vi "Get mode.vi"() -> (3 "Robot Mode":T1)   [LabVIEW 2011]
uses:
  <vilib>/Rock Robotics/WPI/DriverStation/WPI_DriverStationRobotMode.ctl
  <vilib>/Rock Robotics/WPI/DriverStation/WPI_DriverStationCommDataCacheOp.ctl
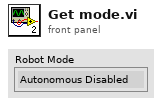
[diagram p1: front panel]
types:
  T1 = typedef "WPI_DriverStationRobotMode.ctl" = enum16{"Autonomous Disabled", "Autonomous Enabled", "Teleop Disabled", "Teleop Enabled", "Timeout", "Finish"}
  T2 = typedef "WPI_DriverStationCommDataCacheOp.ctl" = enum16{"Get", "Set", "Init"}
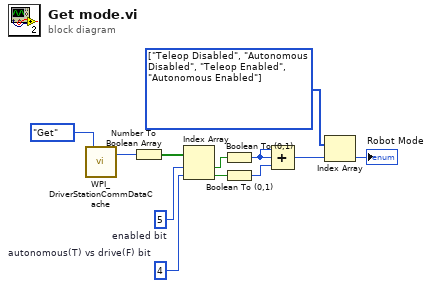
[diagram p0: block diagram]
diagram:
  w7 = T1[] [enum."Teleop Disabled", enum."Autonomous Disabled", enum."Teleop Enabled", enum."Autonomous Enabled"] items=["Autonomous Disabled", "Autonomous Enabled", "Teleop Disabled", "Teleop Enabled", "Timeout", "Finish"]
  w8 = 4  # autonomous(T) vs drive(F) bit
  w9 = 5  # enabled bit
  n1 = call <vilib>:"WPI_DriverStationCommDataCache.vi"("CommDataCacheOp"=WPI_DriverStationCommDataCacheOp."Get") -> ("ControlBit out"=w11:u8)  [unwired: 18 out]
  n2 = Number To Boolean Array(number=w11) -> (Boolean array=w10:bool[])
  n3 = Index Array(array=w10, index #1=w9, index #2=w8) -> (element #1=w4:bool, element #2=w3:bool)
  n4 = Boolean To (0,1)(Boolean=w4) -> (0, 1=w6:i16)
  n5 = Boolean To (0,1)(Boolean=w3) -> (0, 1=w5:i16)
  n6 = Compound Arithmetic op=ADD(w6, w6, w5) -> (w2:i16)
  n7 = Index Array(array=w7, index=w2) -> (element=→"Robot Mode":T1)
